vi "GetType.vi"(8 "error in (no error)":errorcluster, 11 "Configure Measurement Msg":refnum<class "Configure Measurement Msg.lvclass">) -> (0 "error out":errorcluster, 2 "Data Sample":variant, 3 "Configure Measurement Msg":refnum<class "Configure Measurement Msg.lvclass">)   [LabVIEW 2015, in "CS++DMM.lvlib" / "Configure Measurement Msg.lvclass"]
uses:
  Configure Measurement Msg.lvclass
  Configure Measurement Msg.lvclass/Configure Measurement Msg.ctl
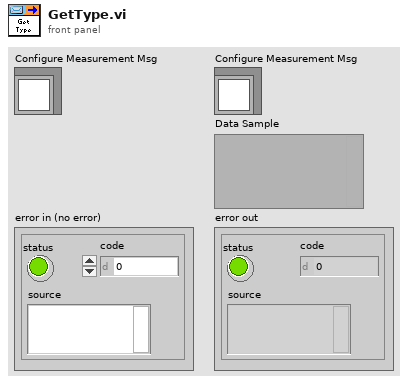
[diagram p1: front panel]
types:
  T1 = cluster{"measurement function (DC Volts)":i32, "absolute resolution (0.001)":dbl, "range (-1.0: Auto)":dbl}
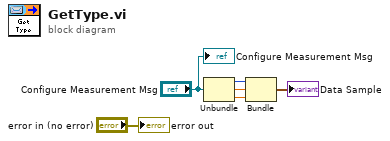
[diagram p0: block diagram]
diagram:
  n1 = Unbundle("Configure Measurement Msg") -> (w3:i32, w2:dbl, w1:dbl)
  n2 = Bundle("measurement function (DC Volts)"=w3, "absolute resolution (0.001)"=w2, "range (-1.0: Auto)"=w1) -> (→"Data Sample":T1)  [unwired: 1 in]
  "error out" <- "error in (no error)"
  "Configure Measurement Msg" <- "Configure Measurement Msg"
